vi "VoltageIO.vi"() -> ()   [LabVIEW 2017]
uses:
  VoltageIO.ctl
  <vilib>/DAQmx/write.llb/DAQmx Write (Analog DBL 1Chan 1Samp).vi
  <vilib>/DAQmx/create/channels.llb/DAQmx Create Channel (AO-Voltage-Basic).vi
  <vilib>/DAQmx/miscellaneous.llb/DAQmx Fill In Error Info.vi
panel:
  in  "physical channels":tag
  in  "stop":bool
  in  "Scrollbar Max (V)":dbl=10.0 min=-10.0 max=10.0
  in  "Scrollbar Min (V)":dbl=-10.0 min=-10.0 max=10.0
  in  "Slide":dbl(slide) min=5.0 max=10.0 step=0.01 scale=5.0..10.0 scale format="%#_6f"
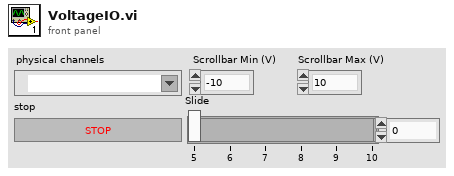
[diagram p1: front panel]
types:
  T1 = typedef "VoltageIO.ctl" = enum16{"Initialize", "Wait for UI", "Update", "Stop"}
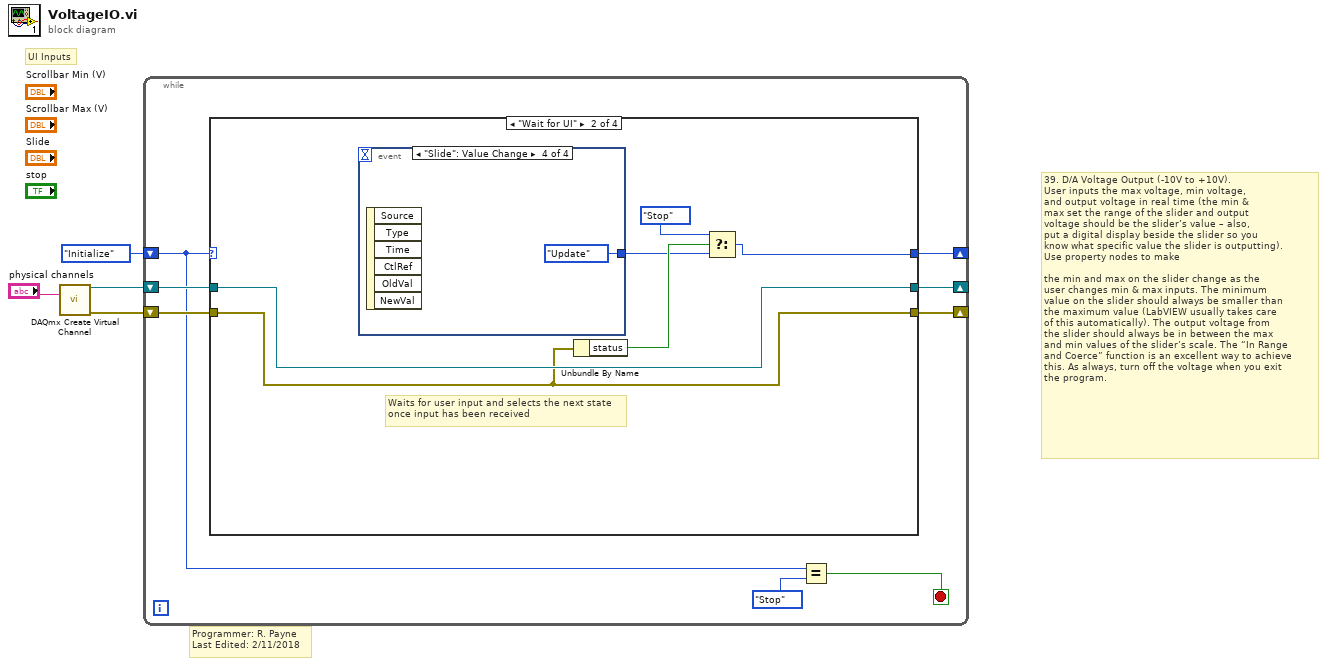
[diagram p0: block diagram]
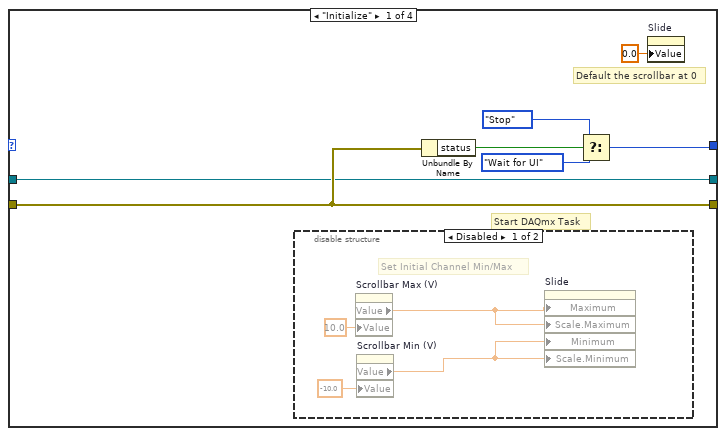
[diagram p2: hidden frame]
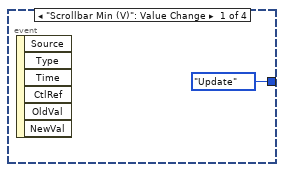
[diagram p4: hidden frame]
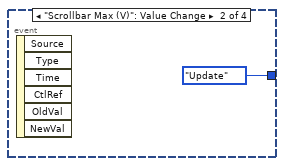
[diagram p5: hidden frame]
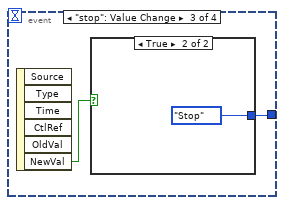
[diagram p6: hidden frame]
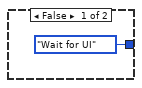
[diagram p7: hidden frame]
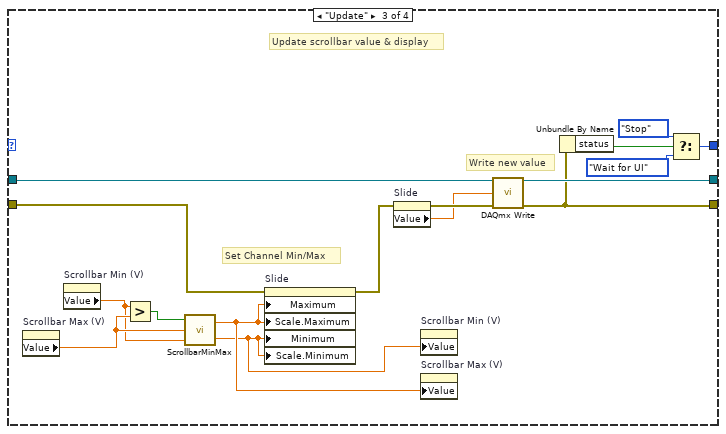
[diagram p8: hidden frame]
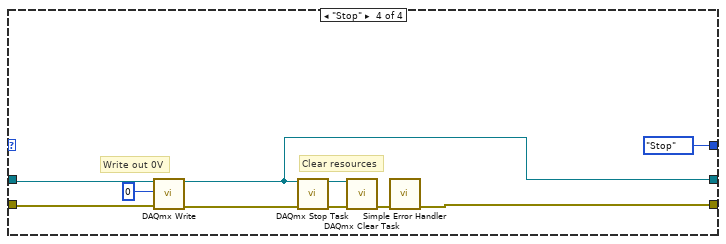
[diagram p9: hidden frame]
diagram:
  # "UI Inputs"
  # "39. D/A Voltage Output (-10V to +10V). \nUser inputs the max voltage, min voltage, \nand output voltage in real time (the min & \nmax set the range of the slider and output \nvoltage should be the slider’s value – also, \nput a digital display beside the slider so you \nknow what specific value the slider is outputting). \nUse property nodes to make\n\nthe min and max on the slider change as the \nuser changes min & max inputs. The minimum \nvalue on the slider should always be smaller than \nthe maximum value (LabVIEW usually takes care \nof this automatically). The output voltage from \nthe slider should always be in between the max \nand min values of the slider’s scale. The “In Range \nand Coerce” function is an excellent way to achieve \nthis. As always, turn off the voltage when you exit \nthe program."
  # "Programmer: R. Payne\nLast Edited: 2/11/2018"
  n1 = call-poly <vilib>:"DAQmx Create Virtual Channel.vi"("physical channels"="physical channels") -> ("task out"=w2:refnum<k21>, "error out"=w1:errorcluster)  [unwired: 13 in]
  n2 = while {
    shift-right: [w12] -> _
    shift-left: VoltageIO."Initialize" -> [w7]
    shift-right: [w11] -> _
    shift-left: w2 -> [w8]
    shift-right: [w10] -> _
    shift-left: w1 -> [w9]
    stop <- w5 stop-if-true
    n3 = case shown="\"Wait for UI\"" w7 {
      tunnel: [w17 w24 w51 VoltageIO."Stop"] -> w12
      tunnel: [w14 w29 w49 w54] -> w11
      tunnel: [w16 w28 w48 w53] -> w10
      tunnel: w9 -> [w16 w28 w41 w58]
      tunnel: w8 -> [w14 w29 w46 w57]
      frame "Initialize" {
        # "Start DAQmx Task"
        # "Default the scrollbar at 0"
        n4 = disable-structure shown="Disabled" {
          frame Disabled {
            # "Set Initial Channel Min/Max"
            n5 = property on="Scrollbar Max (V)" class="DigNum (strict)"("Value"=10.0 ("Scrollbar Max (V)")) -> ("Value"=w21:dbl)  [unwired: 2 in, 2 out]
            n6 = property on="Scrollbar Min (V)" class="DigNum (strict)"("Value"=-10.0 ("Scrollbar Min (V)")) -> ("Value"=w20:dbl)  [unwired: 2 in, 2 out]
            n7 = property on="Slide" class="Slide (strict)"("Maximum"=w21, "Scale.Maximum"=w21, "Minimum"=w20, "Scale.Minimum"=w20) -> ()  [unwired: 2 in, 2 out]
          }
          frame Enabled {
          }
        }
        n8 = Unbundle By Name(w16) -> ("status"=w15:bool)
        n9 = Select(t=VoltageIO."Stop", s=w15, f=VoltageIO."Wait for UI") -> (s? t:f=w17:T1)
        n10 = property on="Slide" class="Slide (strict)"("Value"=0.0 ("Slide")) -> ()  [unwired: 2 in, 2 out]
      }
      frame "Wait for UI" {
        # "Waits for user input and selects the next state\nonce input has been received"
        n11 = event shown="[3] \"Slide\": Value Change" {
          selector: _ -> [_ _ _ _]
          dyn-events: _ -> [_ _ _ _]
          timeout: _ -> [_ _ _ _]
          tunnel: [VoltageIO."Update" VoltageIO."Update" w32 VoltageIO."Update"] -> w26
          event "Scrollbar Min (V)": Value Change {
            n12 = event-data() -> ()  [unwired: 1 in, 6 out]
          }
          event "Scrollbar Max (V)": Value Change {
            n13 = event-data() -> ()  [unwired: 1 in, 6 out]
          }
          event "stop": Value Change {
            n14 = event-data() -> ("NewVal"=w33:bool)  [unwired: 1 in, 5 out]
            n15 = case shown="True" w33 {
              tunnel: [VoltageIO."Wait for UI" VoltageIO."Stop"] -> w32
              frame False {
              }
              frame True {
              }
            }
          }
          event "Slide": Value Change {
            n16 = event-data() -> ()  [unwired: 1 in, 6 out]
          }
        }
        n17 = Unbundle By Name(w28) -> ("status"=w27:bool)
        n18 = Select(t=VoltageIO."Stop", s=w27, f=w26) -> (s? t:f=w24:T1)
      }
      frame "Update" {
        # "Write new value"
        # "Update scrollbar value & display"
        # "Set Channel Min/Max"
        n19 = property on="Scrollbar Max (V)" class="DigNum (strict)"() -> ("Value"=w40:dbl)  [unwired: 2 in, 2 out]
        n20 = property on="Scrollbar Min (V)" class="DigNum (strict)"() -> ("Value"=w39:dbl)  [unwired: 2 in, 2 out]
        n21 = Greater?(x=w39, y=w40) -> (0:w42:bool)
        n22 = call "ScrollbarMinMax.vi"("Scrollbar Min (V) 2"=w39, "Scrollbar Max (V) 2"=w40, "Upper/Lower"=w42) -> ("New Scrollbar Min"=w37:dbl, "New Scrollbar Max"=w38:dbl)
        n23 = property on="Slide" class="Slide (strict)"(error in=w41, "Maximum"=w38, "Scale.Maximum"=w38, "Minimum"=w37, "Scale.Minimum"=w37) -> (error out=w44:errorcluster)  [unwired: 1 in, 1 out]
        n24 = property on="Slide" class="Slide (strict)"(error in=w44) -> (error out=w45:errorcluster, "Value"=w43:dbl)  [unwired: 1 in, 1 out]
        n25 = property on="Scrollbar Min (V)" class="DigNum (strict)"("Value"=w37) -> ()  [unwired: 2 in, 2 out]
        n26 = property on="Scrollbar Max (V)" class="DigNum (strict)"("Value"=w38) -> ()  [unwired: 2 in, 2 out]
        n27 = call-poly <vilib>:"DAQmx Write.vi"("task/channels in"=w46, "data"=w43, "error in"=w45) -> ("task out"=w49:refnum<k21>, "error out"=w48:errorcluster)  [unwired: 10 in, 1 out]
        n28 = Unbundle By Name(w48) -> ("status"=w47:bool)
        n29 = Select(t=VoltageIO."Stop", s=w47, f=VoltageIO."Wait for UI") -> (s? t:f=w51:T1)
      }
      frame "Stop" {
        # "Write out 0V"
        # "Clear resources"
        n30 = call-poly <vilib>:"DAQmx Write.vi"("task/channels in"=w57, "data"=u32 0, "error in"=w58) -> ("task out"=w54:refnum<k21>, "error out"=w60:errorcluster)  [unwired: 10 in, 1 out]
        n31 = call <vilib>:"DAQmx Stop Task.vi"("task/channels in"=w54, "error in"=w60) -> ("task out"=w61:refnum<k21>, "error out"=w62:errorcluster)  [unwired: 12 in]
        n32 = call <vilib>:"DAQmx Clear Task.vi"("task in"=w61, "error in"=w62) -> ("error out"=w55:errorcluster)  [unwired: 13 in]
        n33 = call <vilib>:"Simple Error Handler.vi"("error in (no error)"=w55) -> ("error out"=w53:errorcluster)  [unwired: 4 in, 4 out]
      }
    }
    n34 = Equal?(x=w7, y=VoltageIO."Stop") -> (x = y?=w5:bool)
  }
